vi "Check_Aero_Tunnel_on_Server.vi"(0 "Values":dbl[](array[numeric]) format="%.2f", 2 "Ch Names":string[](array[string]), 3 "Current Time":dbl format="%.2f", 4 "Adam Loop Count":i32) -> (6 "Scan comment":string)   [LabVIEW 2010]
panel:
  in  "Tweak time Down":dbl=100.0
  in  "Sec per delta speed down":dbl=1.75
  out "Reset Integral Term":bool
  in  "Tweak time Up":dbl=50.0
  in  "delta t per delta speed":dbl=0.1
  out "Significant speed change?":bool
  out "Valve Dem Pos":dbl
  out "Tweak in working section demanded temp":dbl
  out "Run Aero Chiller PID?":bool
  in  "Delta Speed greater than":dbl=5.0
  in  "Sec per delta speed up":dbl=0.8
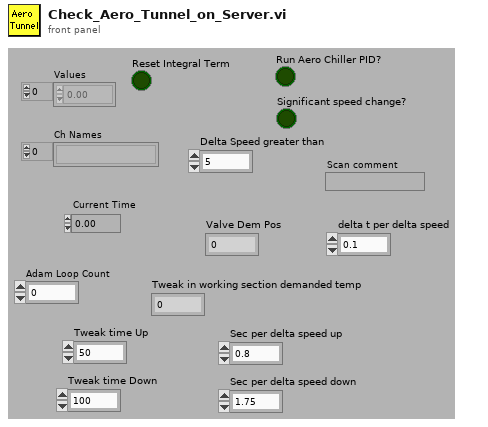
[diagram p1: front panel]
types:
  T1 = typedef "LVDateTimeRec.ctl" = cluster{"fractional second":dbl, "second":i32, "minute":i32, "hour":i32, "day of month":i32, "month":i32, "year":i32, "day of week":i32, "day of year":i32, "DST":i32}
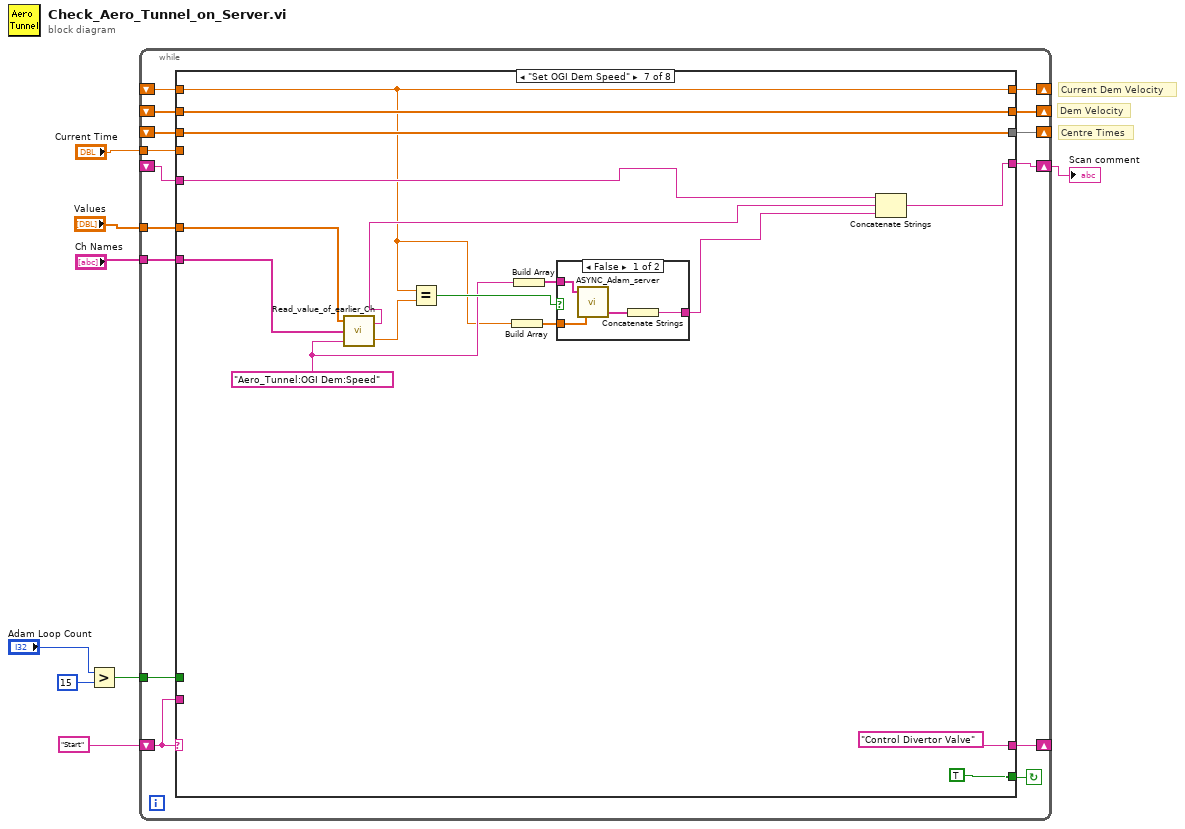
[diagram p0: block diagram]
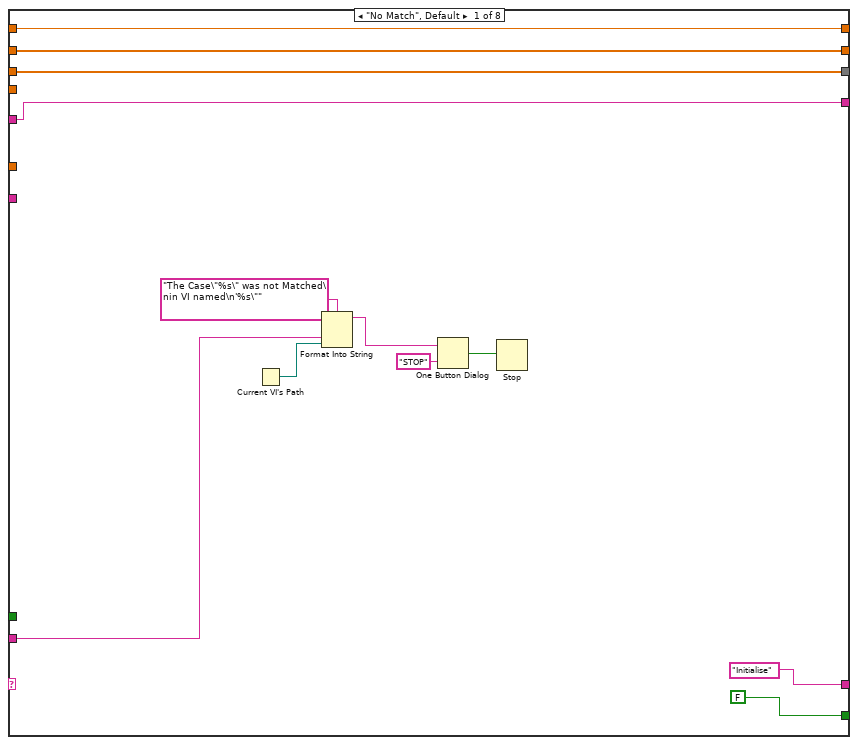
[diagram p2: hidden frame]
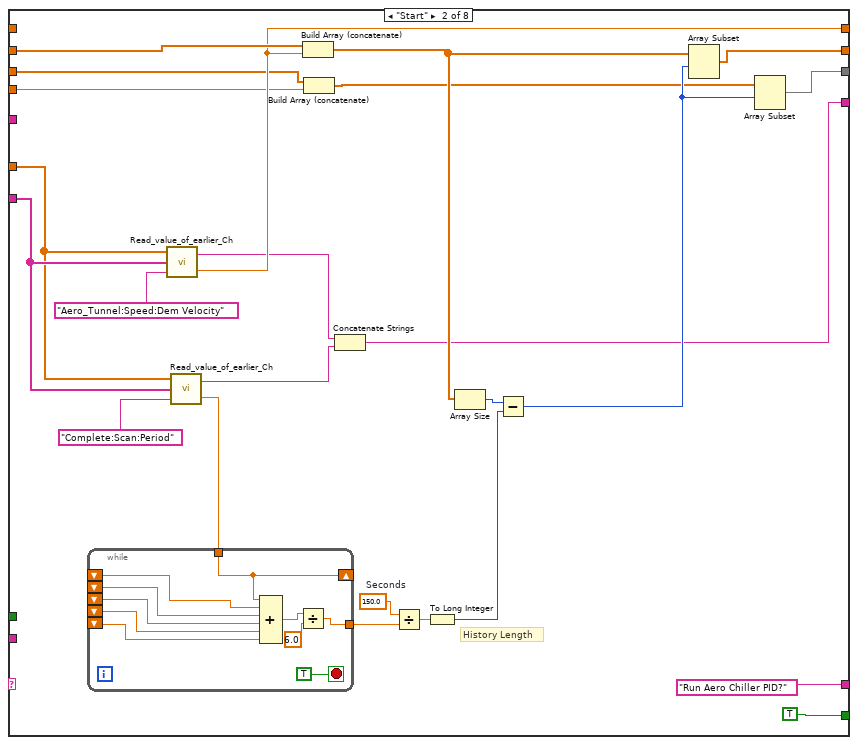
[diagram p3: hidden frame]
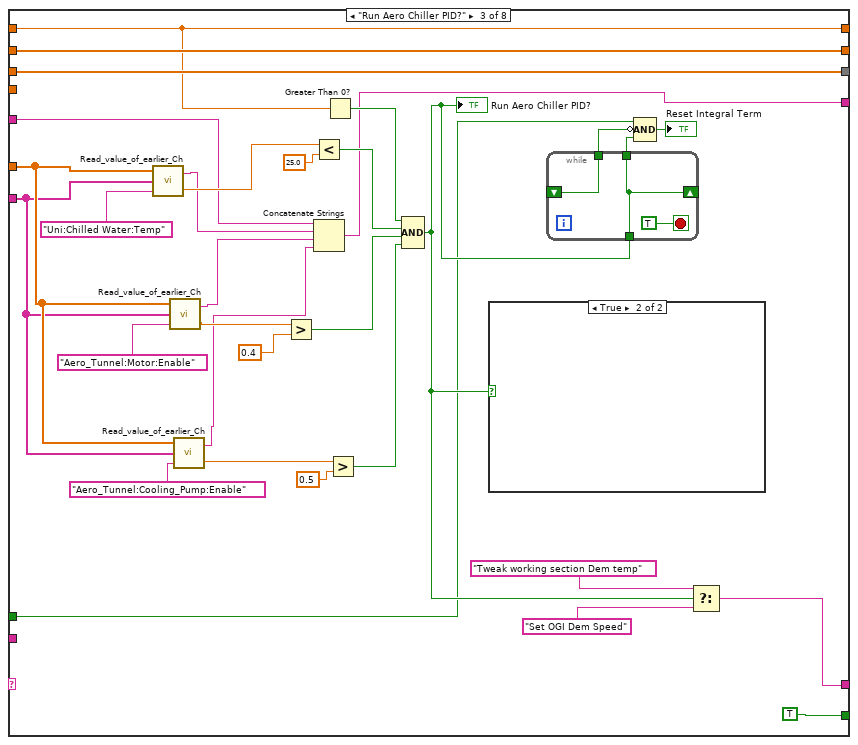
[diagram p4: hidden frame]
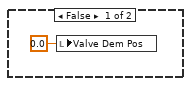
[diagram p5: hidden frame]
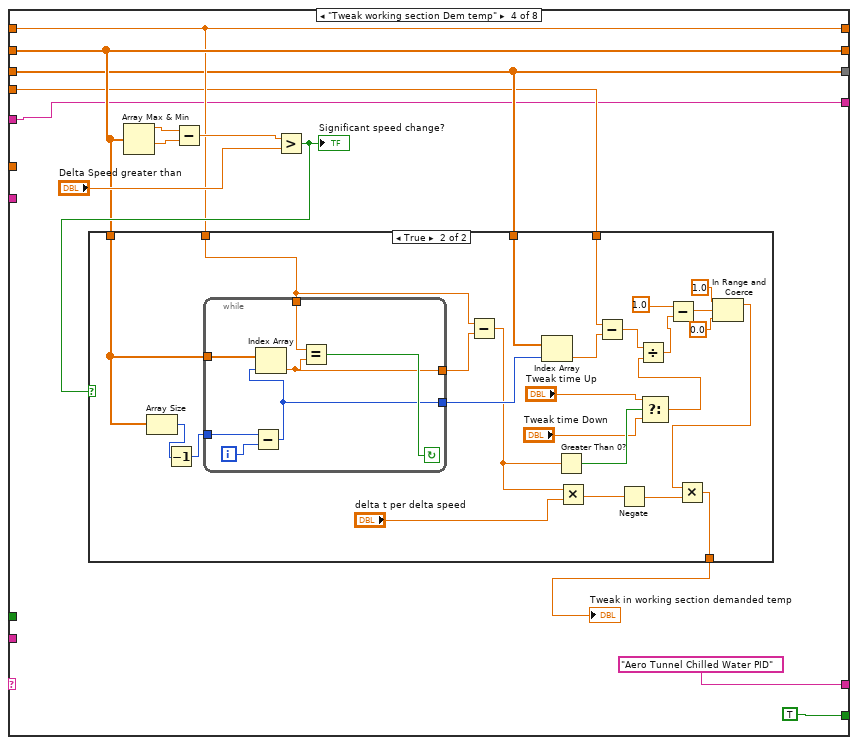
[diagram p6: hidden frame]
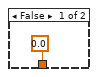
[diagram p7: hidden frame]
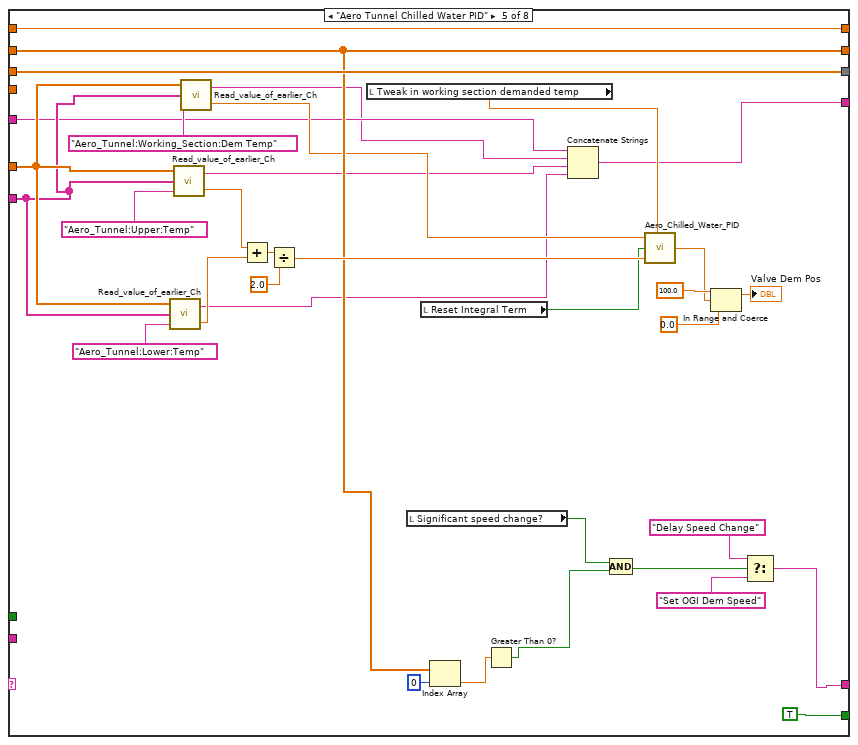
[diagram p8: hidden frame]
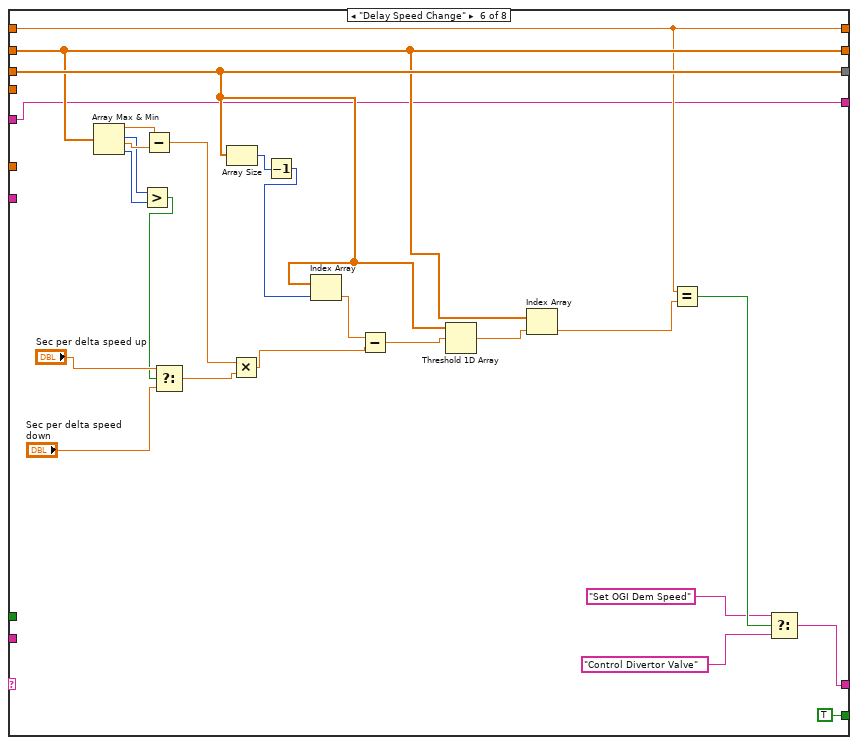
[diagram p9: hidden frame]
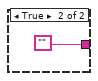
[diagram p10: hidden frame]
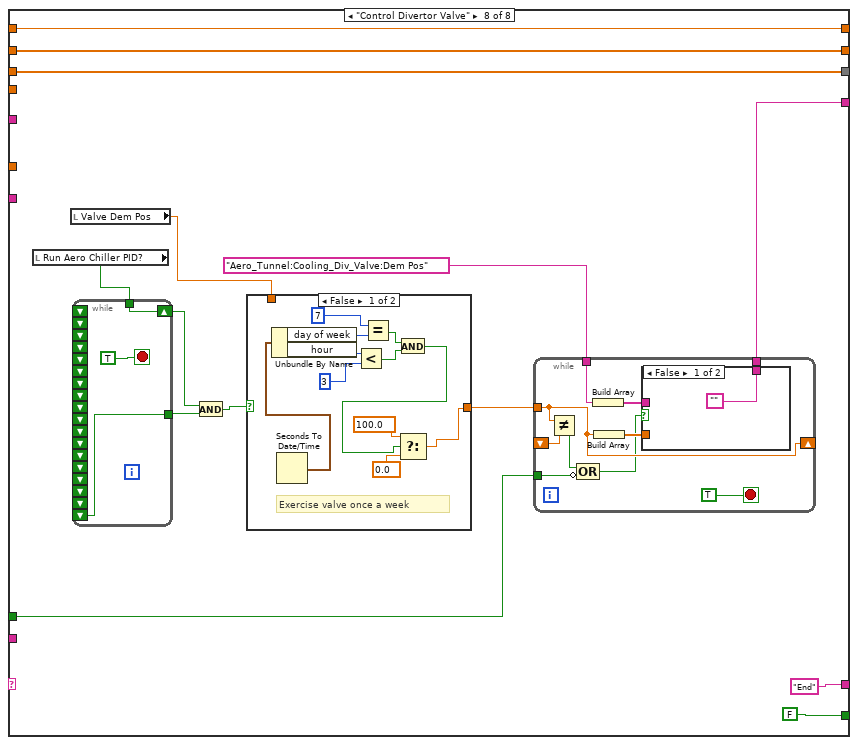
[diagram p11: hidden frame]
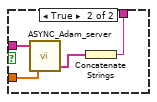
[diagram p13: hidden frame]
diagram:
  # "Dem Velocity"
  # "Centre Times"
  # "Current Dem Velocity"
  n1 = Greater?(x="Adam Loop Count", y=15) -> (0:w2:bool)
  n2 = while {
    shift-left: "Start" -> [w21]
    shift-right: [w22] -> _
    tunnel: "Values" -> [w20]
    tunnel: "Ch Names" -> [w19]
    shift-right: [w18] -> _
    shift-left: _ -> [w17]
    shift-right: [w15] -> _
    shift-left: _ -> [w16]
    shift-right: [w12] -> _
    shift-left: _ -> [w13]
    tunnel: "Current Time" -> [w14]
    tunnel: w2 -> [w11]
    shift-right: [w10] -> w1
    shift-left: _ -> [w9]
    stop <- w23 continue-if-true
    n3 = case shown="\"Set OGI Dem Speed\"" w21 {
      tunnel: [FALSE TRUE TRUE TRUE TRUE TRUE TRUE FALSE] -> w23
      tunnel: ["Initialise" "Run Aero Chiller PID?" ("t") w96 "Aero Tunnel Chilled Water PID" w161 w193 "Control Divertor Valve" "End" ("t")] -> w22
      tunnel: w21 -> [w30 _ _ _ _ _ _ _]
      tunnel: w20 -> [_ w55 w82 _ w171 _ w224 _]
      tunnel: w19 -> [_ w56 w81 _ w170 _ w223 _]
      tunnel: [w27 w50 w87 w110 w181 w200 w212 w242] -> w18
      tunnel: w17 -> [w27 _ w87 w110 w181 w200 w212 w242]
      tunnel: w16 -> [w26 w51 w95 w111 w165 w201 w217 w244]
      tunnel: [w26 w46 w95 w111 w165 w201 w217 w244] -> w15
      tunnel: w14 -> [_ w43 _ w108 _ _ _ _]
      tunnel: w13 -> [w25 w42 w94 w109 w183 w202 w216 w243]
      tunnel: [w25 w40 w94 w109 w183 w202 w216 w243] -> w12
      tunnel: w11 -> [_ _ w76 _ _ _ _ w233]
      tunnel: [w24 w36 w70 w106 w152 w186 w211 w232] -> w10
      tunnel: w9 -> [w24 _ w74 w106 w156 w186 w215 _]
      frame "No Match", Default {
        n4 = Current VI's Path() -> (path=w29:path)
        n5 = Format Into String(format string="The Case\"%s\" was not Matched\nin VI named\n'%s\"" ("Format String"), w30, w29) -> (resulting string=w33:string)  [unwired: 2 in, 1 out]
        n6 = One Button Dialog(message=w33, button name ("OK")="STOP") -> (true=w31:bool)
        n7 = Stop(stop? (T)=w31) -> ()
      }
      frame "Start" {
        w52 = 150.0  # Seconds
        # "History Length"
        n8 = call "Read_value_of_earlier_Ch.vi"("Desired Ch to Read"="Aero_Tunnel:Speed:Dem Velocity", "Ch names"=w56, "Present scan array"=w55) -> ("Value"=w50:dbl, "Scan comment"=w38:string)  [unwired: 1 in]
        n9 = call "Read_value_of_earlier_Ch.vi"("Desired Ch to Read"="Complete:Scan:Period", "Ch names"=w56, "Present scan array"=w55) -> ("Value"=w54:dbl, "Scan comment"=w37:string)  [unwired: 1 in]
        n10 = while {
          shift-right: [w69] -> _
          shift-left: _ -> [w68]
          tunnel: w54 -> [w69]
          shift-left: _ -> [w67]
          shift-left: _ -> [w66]
          shift-left: _ -> [w65]
          shift-left: _ -> [w64]
          tunnel: [w60] -> w53
          stop <- TRUE stop-if-true
          n11 = Compound Arithmetic op=ADD(w69, w68, w67, w66, w65, w64) -> (w62:dbl)
          n12 = Divide(x=w62, y=6.0) -> (x/y=w60:dbl)
        }
        n13 = Build Array (concatenate)(w51, w50) -> (w44:dbl[])
        n14 = Build Array (concatenate)(w42, w43) -> (w41:dbl[])
        n15 = Concatenate Strings(w38, w37) -> (w36:string)
        n16 = Divide(x=w52, y=w53) -> (x/y=w48:dbl)
        n17 = To Long Integer(number=w48) -> (32bit integer=w47:i32)
        n18 = Array Size(array=w44) -> (size(s)=w49:i32)
        n19 = Subtract(x=w49, y=w47) -> (x-y=w45:i32)
        n20 = Array Subset(array=w44, index=w45) -> (w46:dbl[])  [unwired: 1 in]
        n21 = Array Subset(array=w41, index=w45) -> (w40:dbl[])  [unwired: 1 in]
      }
      frame "Run Aero Chiller PID?" {
        n22 = call "Read_value_of_earlier_Ch.vi"("Desired Ch to Read"="Uni:Chilled Water:Temp", "Ch names"=w81, "Present scan array"=w82) -> ("Value"=w99:dbl, "Scan comment"=w73:string)  [unwired: 1 in]
        n23 = call "Read_value_of_earlier_Ch.vi"("Desired Ch to Read"="Aero_Tunnel:Motor:Enable", "Ch names"=w81, "Present scan array"=w82) -> ("Value"=w90:dbl, "Scan comment"=w72:string)  [unwired: 1 in]
        n24 = call "Read_value_of_earlier_Ch.vi"("Desired Ch to Read"="Aero_Tunnel:Cooling_Pump:Enable", "Ch names"=w81, "Present scan array"=w82) -> ("Value"=w84:dbl, "Scan comment"=w71:string)  [unwired: 1 in]
        n25 = Greater?(x=w90, y=0.4) -> (0:w88:bool)
        n26 = Less?(x=w99, y=25.0) -> (x < y?=w89:bool)
        n27 = Concatenate Strings(w74, w73, w72, w71) -> (w70:string)
        n28 = Greater Than 0?(x=w87) -> (x > 0?=w86:bool)
        n29 = Greater?(x=w84, y=0.5) -> (0:w80:bool)
        n30 = Compound Arithmetic op=AND(w86, w89, w88, w80) -> (w79:bool)
        "Run Aero Chiller PID?" <- w79
        n31 = case shown="True" w79 {
          frame False {
            n32 = local write "Valve Dem Pos"(0.0 ("Valve Dem Pos")) -> ()
          }
          frame True {
          }
        }
        n33 = while {
          shift-right: [w103] -> _
          shift-left: _ -> [w104]
          tunnel: w79 -> [w103]
          tunnel: [w104] -> w78
          tunnel: [w103] -> w77
          stop <- TRUE stop-if-true
        }
        n34 = Compound Arithmetic op=AND(w76, invert w78, w77) -> (→"Reset Integral Term":bool)
        n35 = Select(t="Tweak working section Dem temp", s=w79, f="Set OGI Dem Speed") -> (s? t:f=w96:string)
      }
      frame "Tweak working section Dem temp" {
        n36 = Array Max & Min(array=w111) -> (max value=w115:dbl, min value=w116:dbl)  [unwired: 2 out]
        n37 = Subtract(x=w115, y=w116) -> (x-y=w114:dbl)
        n38 = Greater?(x=w114, y="Delta Speed greater than") -> (0:w112:bool)
        "Significant speed change?" <- w112
        n39 = case shown="True" w112 {
          tunnel: w111 -> [_ w143]
          tunnel: w110 -> [_ w137]
          tunnel: w109 -> [_ w140]
          tunnel: w108 -> [_ w139]
          tunnel: [0.0 w127] -> w107
          frame False {
          }
          frame True {
            n40 = Array Size(array=w143) -> (size(s)=w142:i32)
            n41 = Decrement(x=w142) -> (x-1=w144:i32)
            n42 = while {
              tunnel: w144 -> [w150]
              tunnel: w143 -> [w149]
              tunnel: w137 -> [w148]
              tunnel: [w146] -> w141
              tunnel: [w145] -> w136
              i -> [w151]
              stop <- w147 continue-if-true
              n43 = Subtract(x=w150, y=w151) -> (x-y=w146:i32)
              n44 = Index Array(array=w149, index=w146) -> (element=w145:dbl)
              n45 = Equal?(x=w148, y=w145) -> (x = y?=w147:bool)
            }
            n46 = Subtract(x=w137, y=w136) -> (x-y=w124:dbl)
            n47 = Index Array(array=w140, index=w141) -> (element=w138:dbl)
            n48 = Greater Than 0?(x=w124) -> (x > 0?=w123:bool)
            n49 = Multiply(x=w124, y="delta t per delta speed") -> (x*y=w126:dbl)
            n50 = Subtract(x=w139, y=w138) -> (x-y=w133:dbl)
            n51 = Negate(x=w126) -> (-x=w125:dbl)
            n52 = Select(t="Tweak time Up", s=w123, f="Tweak time Down") -> (s? t:f=w120:dbl)
            n53 = Divide(x=w133, y=w120) -> (x/y=w132:dbl)
            n54 = Subtract(x=1.0, y=w132) -> (x-y=w131:dbl)
            n55 = In Range and Coerce(upper limit=1.0, x=w131, lower limit=0.0) -> (coerced(x)=w128:dbl)  [unwired: 1 out]
            n56 = Multiply(x=w128, y=w125) -> (x*y=w127:dbl)
          }
        }
        "Tweak in working section demanded temp" <- w107
      }
      frame "Aero Tunnel Chilled Water PID" {
        n57 = call "Read_value_of_earlier_Ch.vi"("Desired Ch to Read"="Aero_Tunnel:Lower:Temp", "Ch names"=w170, "Present scan array"=w171) -> ("Value"=w174:dbl, "Scan comment"=w153:string)  [unwired: 1 in]
        n58 = call "Read_value_of_earlier_Ch.vi"("Desired Ch to Read"="Aero_Tunnel:Upper:Temp", "Ch names"=w170, "Present scan array"=w171) -> ("Value"=w175:dbl, "Scan comment"=w154:string)  [unwired: 1 in]
        n59 = call "Read_value_of_earlier_Ch.vi"("Desired Ch to Read"="Aero_Tunnel:Working_Section:Dem Temp", "Ch names"=w170, "Present scan array"=w171) -> ("Value"=w157:dbl, "Scan comment"=w155:string)  [unwired: 1 in]
        n60 = Add(x=w175, y=w174) -> (x+y=w176:dbl)
        n61 = Divide(x=w176, y=2.0) -> (x/y=w173:dbl)
        n62 = local read "Tweak in working section demanded temp"() -> (w158:dbl)
        n63 = local read "Significant speed change?"() -> (w160:bool)
        n64 = local read "Reset Integral Term"() -> (w159:bool)
        n65 = Index Array(array=w165, index=0) -> (element=w167:dbl)
        n66 = Greater Than 0?(x=w167) -> (x > 0?=w166:bool)
        n67 = Concatenate Strings(w156, w155, w154, w153) -> (w152:string)
        n68 = Compound Arithmetic op=AND(w160, w166) -> (w162:bool)
        n69 = call "Aero_Chilled_Water_PID.vi"("Tweak in working section demanded temp"=w158, "Present Value"=w173, "Reset PID"=w159, "Setpoint"=w157) -> ("Dem Output"=w178:dbl)
        n70 = In Range and Coerce(upper limit=100.0, x=w178, lower limit=0.0) -> (coerced(x)=→"Valve Dem Pos":dbl)  [unwired: 1 out]
        n71 = Select(t="Delay Speed Change", s=w162, f="Set OGI Dem Speed") -> (s? t:f=w161:string)
      }
      frame "Delay Speed Change" {
        n72 = Array Max & Min(array=w201) -> (max value=w209:dbl, max index (indices)=w192:i32, min value=w210:dbl, min index (indices)=w191:i32)
        n73 = Greater?(x=w192, y=w191) -> (0:w188:bool)
        n74 = Subtract(x=w209, y=w210) -> (x-y=w199:dbl)
        n75 = Select(t="Sec per delta speed up", s=w188, f="Sec per delta speed down") -> (s? t:f=w187:dbl)
        n76 = Array Size(array=w202) -> (size(s)=w204:i32)
        n77 = Multiply(x=w199, y=w187) -> (x*y=w198:dbl)
        n78 = Decrement(x=w204) -> (x-1=w203:i32)
        n79 = Index Array(array=w202, index=w203) -> (element=w205:dbl)
        n80 = Subtract(x=w205, y=w198) -> (x-y=w206:dbl)
        n81 = Threshold 1D Array(2:w206, 3:w202) -> (0:w207:dbl)  [unwired: 1 out]
        n82 = Index Array(array=w201, index=w207) -> (element=w208:dbl)
        n83 = Equal?(x=w200, y=w208) -> (x = y?=w196:bool)
        n84 = Select(t="Set OGI Dem Speed", s=w196, f="Control Divertor Valve") -> (s? t:f=w193:string)
      }
      frame "Set OGI Dem Speed" {
        w220 = "Aero_Tunnel:OGI Dem:Speed"
        n85 = call "Read_value_of_earlier_Ch.vi"("Desired Ch to Read"=w220, "Ch names"=w223, "Present scan array"=w224) -> ("Value"=w222:dbl, "Scan comment"=w214:string)  [unwired: 1 in]
        n86 = Equal?(x=w212, y=w222) -> (x = y?=w221:bool)
        n87 = Build Array(w212) -> (w218:dbl[])
        n88 = Build Array(w220) -> (w219:string[])
        n89 = case shown="False" w221 {
          tunnel: w218 -> [w230 _]
          tunnel: w219 -> [w229 _]
          tunnel: [w227 ""] -> w213
          frame False {
            n90 = call "ASYNC_Adam_server.vi"("Values"=w230, "Channel Names"=w229) -> ("Scan Comments"=w228:string[])  [unwired: 1 in, 2 out]
            n91 = Concatenate Strings(w228) -> (w227:string)
          }
          frame True {
          }
        }
        n92 = Concatenate Strings(w215, w214, w213) -> (w211:string)
      }
      frame "Control Divertor Valve" {
        n93 = local read "Run Aero Chiller PID?"() -> (w235:bool)
        n94 = local read "Valve Dem Pos"() -> (w234:dbl)
        n95 = while {
          shift-right: [w275] -> w236
          shift-left: _ -> [_]
          tunnel: w235 -> [w275]
          shift-left: _ -> [_]
          shift-left: _ -> [_]
          shift-left: _ -> [_]
          shift-left: _ -> [_]
          shift-left: _ -> [_]
          shift-left: _ -> [_]
          shift-left: _ -> [_]
          shift-left: _ -> [_]
          shift-left: _ -> [_]
          shift-left: _ -> [_]
          shift-left: _ -> [_]
          shift-left: _ -> [_]
          shift-left: _ -> [_]
          shift-left: _ -> [_]
          shift-left: _ -> [_]
          shift-left: _ -> [_]
          shift-left: _ -> [w274]
          tunnel: [w274] -> w238
          stop <- TRUE stop-if-true
        }
        n96 = And(x=w236, y=w238) -> (x .and. y?=w239:bool)
        n97 = case shown="False" w239 {
          tunnel: [w247 w257] -> w240
          tunnel: w234 -> [_ w257]
          frame False {
            # "Exercise valve once a week"
            n98 = Seconds To Date/Time() -> (date time rec=w248:T1)  [unwired: 2 out]
            n99 = Unbundle By Name(w248) -> ("day of week"=w253:i32, "hour"=w251:i32)
            n100 = Less?(x=w251, y=3) -> (x < y?=w256:bool)
            n101 = Equal?(x=7, y=w253) -> (x = y?=w255:bool)
            n102 = And(x=w255, y=w256) -> (x .and. y?=w246:bool)
            n103 = Select(t=100.0, s=w246, f=0.0) -> (s? t:f=w247:dbl)
          }
          frame True {
          }
        }
        n104 = while {
          shift-right: [w263] -> _
          shift-left: _ -> [w264]
          tunnel: w240 -> [w263]
          tunnel: "Aero_Tunnel:Cooling_Div_Valve:Dem Pos" -> [w265]
          tunnel: w233 -> [w260]
          tunnel: [w258] -> w232
          stop <- TRUE stop-if-true
          n105 = Not Equal?(x=w263, y=w264) -> (x != y?=w261:bool)
          n106 = Compound Arithmetic op=OR(w261, invert w260) -> (w259:bool)
          n107 = Build Array(w265) -> (w266:string[])
          n108 = Build Array(w263) -> (w267:dbl[])
          n109 = case shown="False" w259 {
            tunnel: w267 -> [_ w272]
            tunnel: w266 -> [_ w271]
            tunnel: ["" w269] -> w258
            frame False {
            }
            frame True {
              n110 = call "ASYNC_Adam_server.vi"("Values"=w272, "Channel Names"=w271) -> ("Scan Comments"=w270:string[])  [unwired: 1 in, 2 out]
              n111 = Concatenate Strings(w270) -> (w269:string)
            }
          }
        }
      }
    }
  }
  "Scan comment" <- w1
